vi "Launcher.vi"   [LabVIEW 2025]
uses:
  Application/Application Manager/Application Manager/Application Manager.lvclass
  <vilib>/Natan Biesmans/G2CPU GPU and CPU HPC Toolkit/G2CPU Libraries/Runtime Licensing/G2CPU License Check.vi
  <vilib>/Natan Biesmans/G2CPU GPU and CPU HPC Toolkit/ArrayFire Driver/VIs/init.vi
  <vilib>/Natan Biesmans/G2CPU GPU and CPU HPC Toolkit/G2CPU Libraries/Async IO/CUDA Context FGV.vi
  <resource>/Natan Biesmans/G2CPU GPU and CPU HPC Toolkit/Garbage Collector/G2CPU GarbageCollectorFGV.vi
  <resource>/Natan Biesmans/G2CPU GPU and CPU HPC Toolkit/Garbage Collector/G2CPU DMAGarbageCollectorFGV.vi
  <vilib>/ActorFramework/Actor/Actor.lvclass
  <vilib>/MGI/Monitored Actor/Monitored Actor.lvlib
panel:
  # "Launching, Please wait."
types:
  T1 = enum32{"Invalid", "Standard", "Closed", "Hidden", "Minimized", "Maximized"}
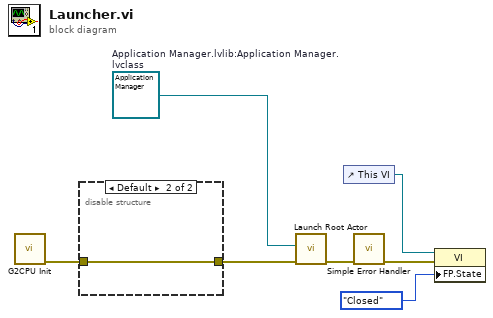
[diagram p0: block diagram]
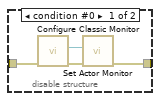
[diagram p2: hidden frame]
diagram:
  w1 = refnum<class "Application Manager.lvclass"> refnum  # Application Manager.lvlib:Application Manager.lvclass
  n1 = call <vilib>:"G2CPU Init.vi"() -> ("error out"=w2:errorcluster)  [unwired: 11 in]
  n2 = disable-structure shown="Default" {
    disable-tunnel: [w9 w12] -> w6
    disable-tunnel: w2 -> [w8 w12]
    frame condition #0 {
      n3 = call <vilib>:"Configure Classic Monitor.vi"("error in (no error)"=w8) -> ("error out"=w10:errorcluster, "Classic Monitor out"=w11:refnum<class "Actor Monitor.lvclass">)  [unwired: 9 in]
      n4 = call <vilib>:"Set Actor Monitor.vi"("error in (no error)"=w10, "Actor Monitor"=w11) -> ("error out"=w9:errorcluster)  [unwired: 9 in]
    }
    frame condition #1 (active) {
    }
  }
  n5 = call <vilib>:"Launch Root Actor.vi"("error in (no error)"=w6, "Actor"=w1) -> ("error out"=w7:errorcluster)  [unwired: 8 in, 1 out]
  n6 = control-ref of="This VI"() -> (w4:refnum<vi>)
  n7 = call <vilib>:"Simple Error Handler.vi"("error in (no error)"=w7) -> ("error out"=w5:errorcluster)  [unwired: 4 in, 4 out]
  n8 = property class="VI"(reference=w4, error in=w5, "FP.State"=T1."Closed" ("Front Panel Window:State")) -> ()  [unwired: 2 out]
